vi "Refresh.vi"(8 "error in (no error)":errorcluster, 11 "Main in":refnum<class "Main.lvclass">) -> (0 "error out":errorcluster, 3 "Main out":refnum<class "Main.lvclass">)   [LabVIEW 2020, in "Main.lvclass"]
uses:
  Main.lvclass
  Debugger/Debugger.lvclass
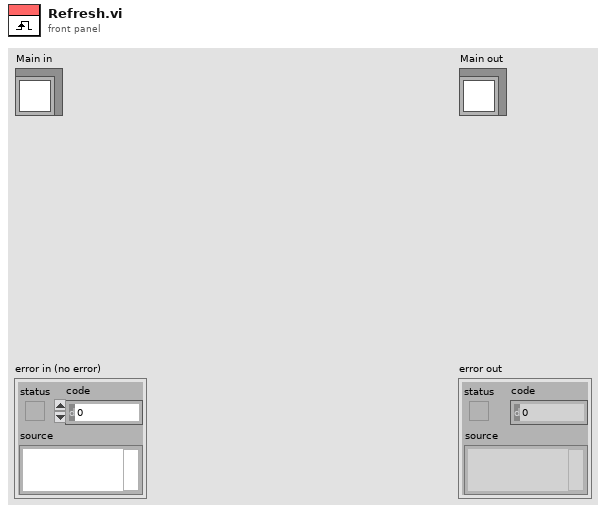
[diagram p1: front panel]
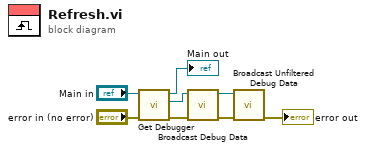
[diagram p0: block diagram]
diagram:
  n1 = call "Get Debugger.vi"("error in (no error)"="error in (no error)", "Main In"="Main in") -> ("error out"=w4:errorcluster, "Debugger.lvclass"=w6:refnum<class "Debugger.lvclass">, "Main Out"=→"Main out":refnum<class "Main.lvclass">)  [unwired: 7 in]
  n2 = call "Broadcast Debug Data.vi"("error in (no error)"=w4, "Debugger in"=w6) -> ("error out"=w3:errorcluster, "Debugger out"=w5:refnum<class "Debugger.lvclass">)  [unwired: 8 in]
  n3 = call "Broadcast Unfiltered Debug Data.vi"("error in (no error)"=w3, "Debugger in"=w5) -> ("error out"=→"error out":errorcluster)  [unwired: 8 in, 1 out]
